vi "Right Side Drive.vi"(11 "Effort":dbl=-0.007874015748031496) -> ()   [LabVIEW 2017]
uses:
  <vilib>/Rock Robotics/WPI/ThirdParty/Phoenix-LabVIEW/Motor Controller/Controls/CTRE_Phoenix_MotorControl_ControlMode.ctl
  <vilib>/Rock Robotics/WPI/ThirdParty/Phoenix-LabVIEW/Motor Controller/Get/CTRE_Phoenix_MotorController_GetVoltage.vi
panel:
  out "Percent Output right true":dbl
  out "Percent Output Right":dbl
  in  "Min Joystick":dbl=0.1 format="%#_13g"
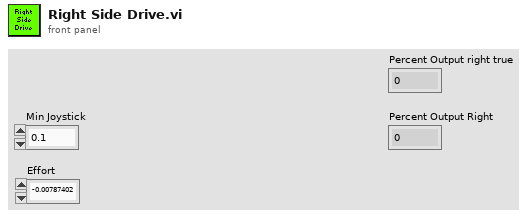
[diagram p1: front panel]
types:
  T1 = typedef "CTRE_Phoenix_MotorControl_ControlMode.ctl" = u16
  T2 = typedef "WPI_MotorControlDeviceRef.ctl" = cluster{"DeviceStatus":errorcluster, "Type":T3, "PWM":cluster{"PWM Channel":T4, "DeadBand":T5}, "CAN":cluster{"Device Number":u8, "SetOutput VI Ref":variant, "GetOutput VI Ref":variant, "Enable VI Ref":variant, "Disable VI Ref":variant, "Data":variant}, "Invert":bool, "DIO PWM":cluster{"PWM \"Enable\" Channel":T4, "DIOChannel":T6, "PWM Rate":dbl}}
  T3 = typedef "WPI_MotorControlType.ctl" = enum16{"PWM", "CAN", "DIO PWM"}
  T4 = typedef "FPGA_DIOPWMChannel.ctl" = enum8{"PWM 0", "PWM 1", "PWM 2", "PWM 3", "PWM 4", "PWM 5", "PWM 6", "PWM 7", "PWM 8", "PWM 9", "PWM MXP 0", "PWM MXP 1", "PWM MXP 2", "PWM MXP 3", "PWM MXP 4", "PWM MXP 5", "PWM MXP 6", "PWM MXP 7", "PWM MXP 8", "PWM MXP 9", "Invalid"}
  T5 = typedef "WPI_PWMDeadband.ctl" = cluster{"Name":string, "maxPositivePwm":i32, "minPositivePwm":i32, "centerPwm":i32, "maxNegativePwm":i32, "minNegativePwm":i32, "angularRange":u16}
  T6 = typedef "FPGA_DIOChannel.ctl" = enum8{"DIO 0", "DIO 1", "DIO 2", "DIO 3", "DIO 4", "DIO 5", "DIO 6", "DIO 7", "DIO 8", "DIO 9", "DIO MXP 0", "DIO MXP 1", "DIO MXP 2", "DIO MXP 3", "DIO MXP 4", "DIO MXP 5", "DIO MXP 6", "DIO MXP 7", "DIO MXP 8", "DIO MXP 9", "DIO MXP 10", "DIO MXP 11", "DIO MXP 12", "DIO MXP 13", "DIO MXP 14", "DIO MXP 15", "SPI Port CS1", "SPI Port CS2", "SPI Port CS3", "SPI Port MISO", "SPI Port MOSI", "Invalid"}
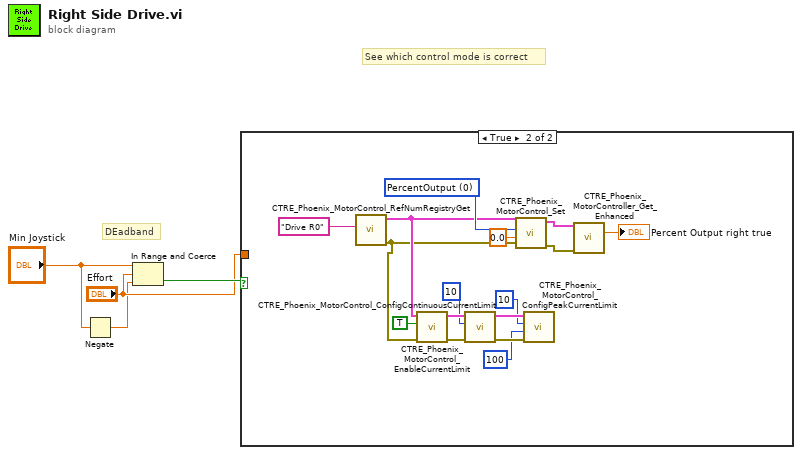
[diagram p0: block diagram]
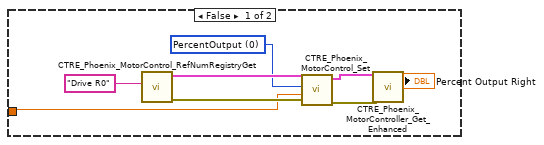
[diagram p2: hidden frame]
diagram:
  # "DEadband"
  # "See which control mode is correct"
  n1 = Negate(x="Min Joystick") -> (-x=w1:dbl)
  n2 = In Range and Coerce(upper limit="Min Joystick", x="Effort", lower limit=w1) -> (In Range?=w4:bool)  [unwired: 1 out]
  n3 = case shown="True" w4 {
    tunnel: "Effort" -> [w8 _]
    frame False {
      w9 = T1 0 items=["PercentOutput"=0, "Position"=1, "Velocity"=2, "Current"=3, "Follower"=5, "MotionProfile"=6, "MotionMagic"=7, "MotionMagicArc"=8, "MotionProfileArc"=10, "Disabled"=15] ("Control Mode")
      n4 = call <vilib>:"CTRE_Phoenix_MotorControl_RefNumRegistryGet.vi"("refnum name"="Drive R0") -> ("error out"=w12:errorcluster, "PhoenixMotorControlDevRef"=w11:T2)  [unwired: 9 in]
      n5 = call <vilib>:"CTRE_Phoenix_MotorControl_Set.vi"("error in (no error)"=w12, "Output"=w8, "Control Mode"=w9, "PhoenixMotorControlDevRef"=w11) -> ("error out"=w6:errorcluster, "PhoenixMotorControlDevRef"=w7:T2)  [unwired: 6 in]
      n6 = call-poly <vilib>:"CTRE_Phoenix_MotorController_Get_Enhanced.vi"("PhoenixMotorControlDevRef"=w7, "error in"=w6) -> ("Percent Output"=→"Percent Output Right":dbl)  [unwired: 9 in, 4 out]
    }
    frame True {
      w27 = T1 0 items=["PercentOutput"=0, "Position"=1, "Velocity"=2, "Current"=3, "Follower"=5, "MotionProfile"=6, "MotionMagic"=7, "MotionMagicArc"=8, "MotionProfileArc"=10, "Disabled"=15] ("Control Mode")
      n7 = call <vilib>:"CTRE_Phoenix_MotorControl_RefNumRegistryGet.vi"("refnum name"="Drive R0") -> ("error out"=w13:errorcluster, "PhoenixMotorControlDevRef"=w14:T2)  [unwired: 9 in]
      n8 = call <vilib>:"CTRE_Phoenix_MotorControl_EnableCurrentLimit.vi"("error in (no error)"=w13, "Enable Current Limit?"=TRUE, "PhoenixMotorControlDevRef"=w14) -> ("error out"=w21:errorcluster, "PhoenixMotorControlDevRef"=w20:T2)  [unwired: 7 in]
      n9 = call <vilib>:"CTRE_Phoenix_MotorControl_ConfigContinuousCurrentLimit.vi"("error in (no error)"=w21, "Continuous Current Limit (Amps)"=10, "PhoenixMotorControlDevRef"=w20) -> ("error out"=w17:errorcluster, "PhoenixMotorControlDevRef"=w18:T2)  [unwired: 7 in]
      n10 = call <vilib>:"CTRE_Phoenix_MotorControl_Set.vi"("error in (no error)"=w13, "Output"=0.0, "Control Mode"=w27, "PhoenixMotorControlDevRef"=w14) -> ("error out"=w23:errorcluster, "PhoenixMotorControlDevRef"=w24:T2)  [unwired: 6 in]
      n11 = call <vilib>:"CTRE_Phoenix_MotorControl_ConfigPeakCurrentLimit.vi"("error in (no error)"=w17, "Peak Current Maximum Duration (ms)"=100, "Peak Current (Amps)"=10, "PhoenixMotorControlDevRef"=w18) -> ()  [unwired: 6 in, 2 out]
      n12 = call-poly <vilib>:"CTRE_Phoenix_MotorController_Get_Enhanced.vi"("PhoenixMotorControlDevRef"=w24, "error in"=w23) -> ("Percent Output"=→"Percent Output right true":dbl)  [unwired: 9 in, 4 out]
    }
  }
